vi "CVT Bool Write.vi"(3 "error in (no error)":errorcluster, 4 "Value":bool, 5 "Tag Name":string) -> (0 "error out":errorcluster)   [LabVIEW 2014, in "QwaveSys Raspberry Pi Library.lvlib"]
uses:
  _SubVIs/TypeDefs/cvt_TagList Methods.ctl
  _SubVIs/TypeDefs/cvt_MemBlock Methods.ctl
  QwaveSys Raspberry Pi Library.lvlib
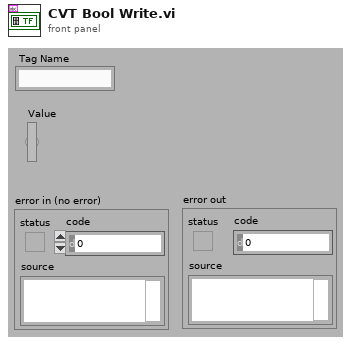
[diagram p1: front panel]
types:
  T1 = typedef "QwaveSys Raspberry Pi Library.lvlib/cvt_MemBlock Methods.ctl" = enum16{"init", "read", "readall", "write"}
  T2 = typedef "QwaveSys Raspberry Pi Library.lvlib/cvt_TagList Methods.ctl" = enum16{"init", "getindex", "getdesc", "getlist"}
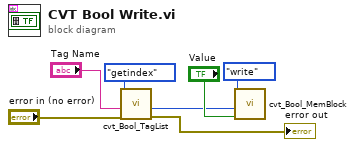
[diagram p0: block diagram]
diagram:
  n1 = call "cvt_Bool_TagList.vi"("error in (no error)"="error in (no error)", "Tag Name"="Tag Name", "Method"=cvt_TagList_Methods."getindex") -> ("error out"=→"error out":errorcluster, "Tag Index"=w5:i32)  [unwired: 1 in, 6 out]
  n2 = call "cvt_Bool_MemBlock.vi"("Value"="Value", "Index"=w5, "Method"=cvt_MemBlock_Methods."write") -> ()  [unwired: 2 in, 7 out]
